vi "SubVI_IntakeArmToggle_TeleOp.vi"(8 "error in (no error)":errorcluster, 11 "Open/Close Intake":bool) -> (0 "error out":errorcluster, 2 "IntakeSolenoid2":T1={"DevStatus"={"status"=FALSE, "code"=0, "source"=""}, "Pneumatics Control Module"=0, "Forward Solenoid Channel"=enum."Invalid", "Reverse Solenoid Channel"=enum."Invalid"}, 3 "IntakeSolenoid1":T1={"DevStatus"={"status"=FALSE, "code"=0, "source"=""}, "Pneumatics Control Module"=0, "Forward Solenoid Channel"=enum."Invalid", "Reverse Solenoid Channel"=enum."Invalid"})   [LabVIEW 2017]
uses:
  <vilib>/Rock Robotics/WPI/Solenoid/WPI_SolenoidDevRef.ctl
  <vilib>/Rock Robotics/WPI/Solenoid/WPI_SolenoidChannel.ctl
  <vilib>/Rock Robotics/WPI/Solenoid/WPI_SolenoidValue.ctl
  <vilib>/Rock Robotics/WPI/Solenoid/WPI_SolenoidSetEnum.vi
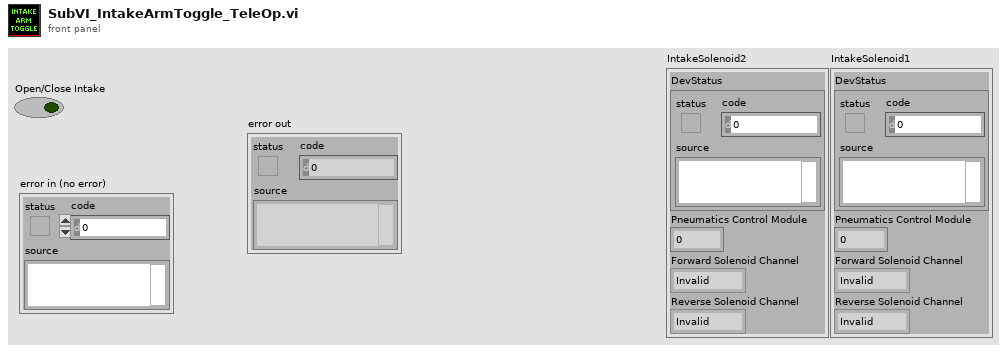
[diagram p1: front panel]
types:
  T1 = typedef "WPI_SolenoidDevRef.ctl" = cluster{"DevStatus":errorcluster, "Pneumatics Control Module":u8, "Forward Solenoid Channel":T2, "Reverse Solenoid Channel":T2}
  T2 = typedef "WPI_SolenoidChannel.ctl" = enum8{"Solenoid 0", "Solenoid 1", "Solenoid 2", "Solenoid 3", "Solenoid 4", "Solenoid 5", "Solenoid 6", "Solenoid 7", "Invalid"}
  T3 = typedef "WPI_SolenoidValue.ctl" = enum16{"Off", "On", "Forward", "Reverse"}
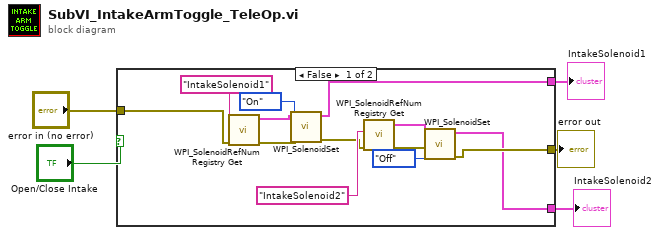
[diagram p0: block diagram]
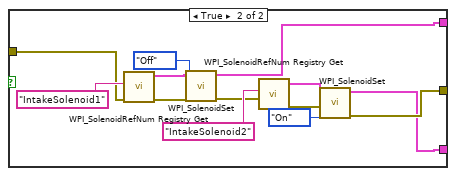
[diagram p2: hidden frame]
diagram:
  n1 = case shown="False" "Open/Close Intake" {
    tunnel: [w9 w21] -> w4
    tunnel: "error in (no error)" -> [w8 w25]
    tunnel: [w7 w20] -> w2
    tunnel: [w6 w19] -> w1
    frame False {
      n2 = call <vilib>:"WPI_SolenoidRefNum Registry Get.vi"("error in (no error)"=w8, "refnum name"="IntakeSolenoid1") -> ("error out"=w12:errorcluster, "SolenoidDevRef"=w18:T1)  [unwired: 8 in]
      n3 = call-poly <vilib>:"WPI_SolenoidSet.vi"("error in (no error)"=w12, "Value"=WPI_SolenoidValue."On", "SolenoidDevRef"=w18) -> ("error out"=w11:errorcluster, "SolenoidDevRef"=w6:T1)  [unwired: 7 in]
      n4 = call <vilib>:"WPI_SolenoidRefNum Registry Get.vi"("error in (no error)"=w11, "refnum name"="IntakeSolenoid2" ("IntakeSolenoid2")) -> ("error out"=w10:errorcluster, "SolenoidDevRef"=w16:T1)  [unwired: 8 in]
      n5 = call-poly <vilib>:"WPI_SolenoidSet.vi"("error in (no error)"=w10, "Value"=WPI_SolenoidValue."Off", "SolenoidDevRef"=w16) -> ("error out"=w9:errorcluster, "SolenoidDevRef"=w7:T1)  [unwired: 7 in]
    }
    frame True {
      n6 = call <vilib>:"WPI_SolenoidRefNum Registry Get.vi"("error in (no error)"=w25, "refnum name"="IntakeSolenoid1") -> ("error out"=w24:errorcluster, "SolenoidDevRef"=w31:T1)  [unwired: 8 in]
      n7 = call-poly <vilib>:"WPI_SolenoidSet.vi"("error in (no error)"=w24, "Value"=WPI_SolenoidValue."Off", "SolenoidDevRef"=w31) -> ("error out"=w23:errorcluster, "SolenoidDevRef"=w19:T1)  [unwired: 7 in]
      n8 = call <vilib>:"WPI_SolenoidRefNum Registry Get.vi"("error in (no error)"=w23, "refnum name"="IntakeSolenoid2") -> ("error out"=w22:errorcluster, "SolenoidDevRef"=w29:T1)  [unwired: 8 in]
      n9 = call-poly <vilib>:"WPI_SolenoidSet.vi"("error in (no error)"=w22, "Value"=WPI_SolenoidValue."On", "SolenoidDevRef"=w29) -> ("error out"=w21:errorcluster, "SolenoidDevRef"=w20:T1)  [unwired: 7 in]
    }
  }
  "error out" <- w4
  "IntakeSolenoid2" <- w2
  "IntakeSolenoid1" <- w1
